vi "UI Initialize.vi"(8 "error in (no error)":errorcluster, 11 "New Project Wizard in":refnum<class "New Project Wizard.lvclass">) -> (0 "error out":errorcluster, 3 "New Project Wizard out":refnum<class "New Project Wizard.lvclass">)   [LabVIEW 2013, in "SET Project Editor.lvlib" / "New Project Wizard.lvclass"]
uses:
  New Project Wizard.lvclass
  New Project Wizard.lvclass/New Project Wizard.ctl
  UI Wizard/UI Wizard.lvclass
  SET Project Editor.lvlib
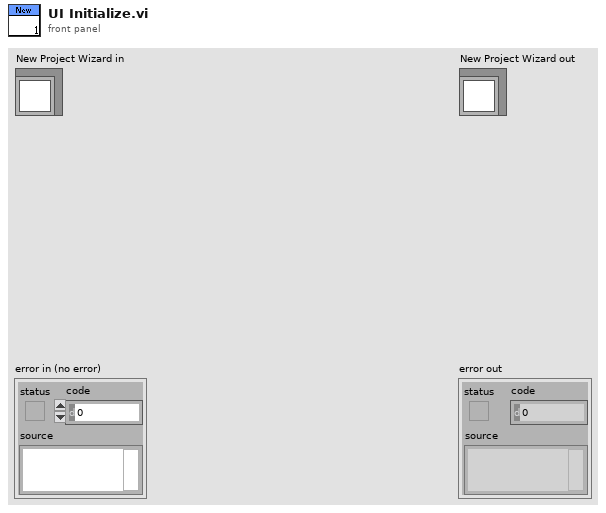
[diagram p1: front panel]
types:
  T1 = enum32{"Invalid", "Default", "Floating", "Floating/Auto-Hide", "Modal"}
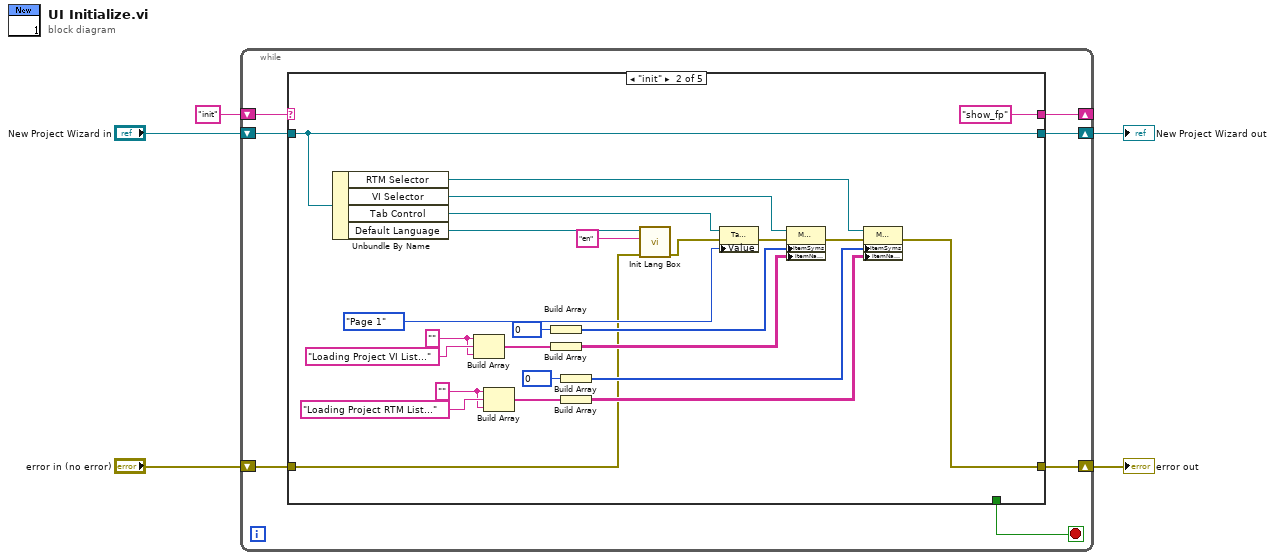
[diagram p0: block diagram]
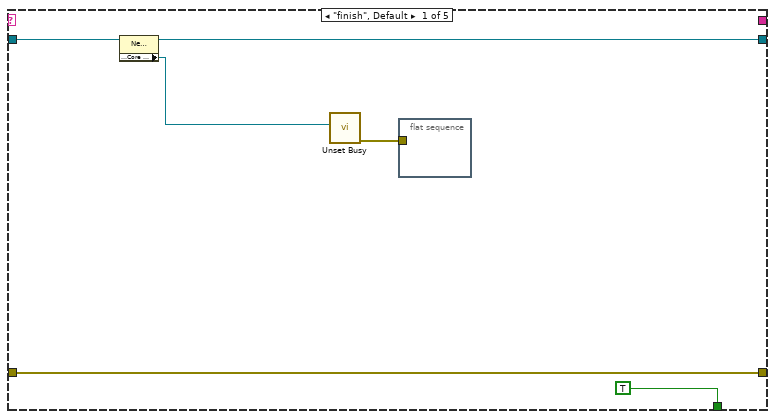
[diagram p2: hidden frame]
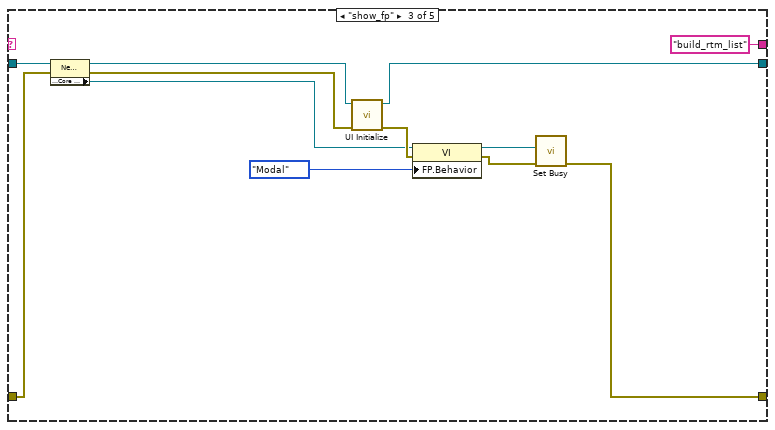
[diagram p3: hidden frame]
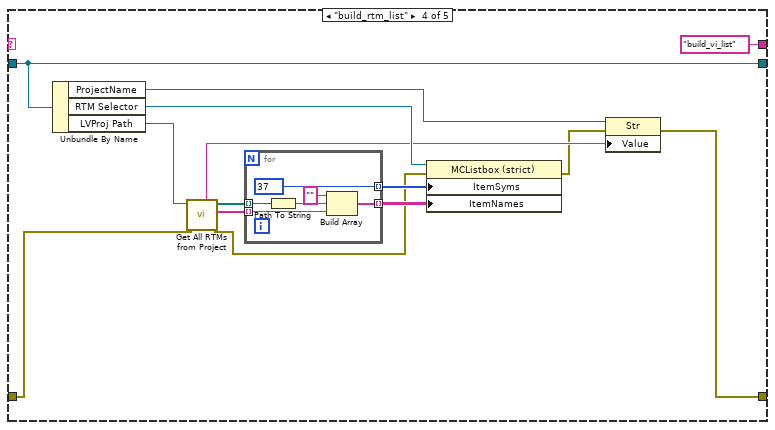
[diagram p4: hidden frame]
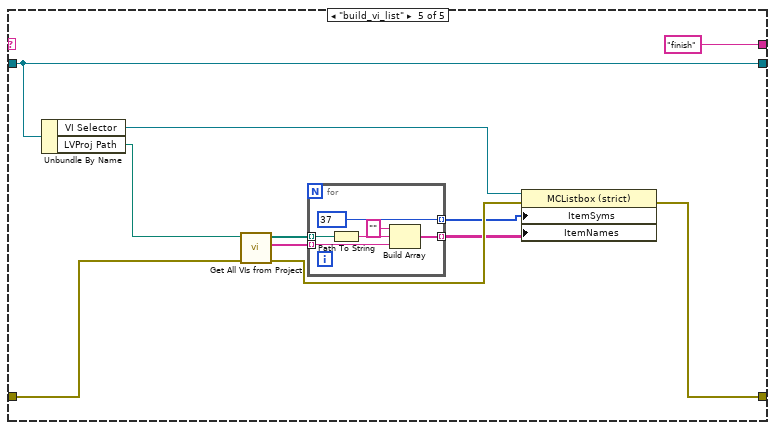
[diagram p5: hidden frame]
diagram:
  n1 = while {
    shift-right: [w8] -> w1
    shift-left: "New Project Wizard in" -> [w12]
    shift-right: [w7] -> _
    shift-left: "init" -> [w11]
    shift-right: [w9] -> w2
    shift-left: "error in (no error)" -> [w10]
    stop <- w6 stop-if-true
    n2 = case shown="\"init\"" w11 {
      tunnel: w12 -> [w16 w24 w53 w59 w77]
      tunnel: w10 -> [w18 w21 w50 w64 w78]
      tunnel: [w18 w25 w45 w57 w81] -> w9
      tunnel: [w15 w24 w48 w59 w77] -> w8
      tunnel: [_ "show_fp" "build_rtm_list" "build_vi_list" "finish"] -> w7
      tunnel: [TRUE _ _ _ _] -> w6
      frame "finish", Default {
        n3 = property class="New Project Wizard.lvclass"(reference=w16) -> (reference out=w15:refnum<class "New Project Wizard.lvclass">, "Properties:Core VI Refnum"=w14:refnum<vi>)  [unwired: 1 in, 1 out]
        n4 = call <vilib>:"Unset Busy.vi"("VI reference (current VI)"=w14) -> ("error out"=w17:errorcluster)  [unwired: 10 in]
        n5 = flat-sequence {
          tunnel: w17 -> [_]
          frame #0 {
          }
        }
      }
      frame "init" {
        w32 = ""
        w38 = ""
        n6 = Unbundle By Name(w24) -> ("RTM Selector"=w29:refnum<vi>, "VI Selector"=w37:refnum<vi>, "Tab Control"=w42:refnum<vi>, "Default Language"=w22:refnum<vi>)
        n7 = Build Array(w38, "Loading Project VI List...", w38) -> (w41:string[])
        n8 = Build Array(w32, "Loading Project RTM List...", w32) -> (w34:string[])
        n9 = Build Array(0) -> (w31:i32[])
        n10 = Build Array(w41) -> (w30:string[][])
        n11 = Build Array(0) -> (w28:i32[])
        n12 = Build Array(w34) -> (w27:string[][])
        n13 = call "Init Lang Box.vi"("error in (no error)"=w21, "Initial Value"="en", "ComboBox Ref in"=w22) -> ("error out"=w19:errorcluster)  [unwired: 7 in, 1 out]
        n14 = property class="TabCtl (strict)"(reference=w42, error in=w19, "Value"=enum32{"Page 1", "Page 2"}."Page 1") -> (error out=w36:errorcluster)  [unwired: 1 out]
        n15 = property on="Property Node" class="MCListbox (strict)"(reference=w37, error in=w36, "ItemSyms"=w31, "ItemNames"=w30) -> (error out=w26:errorcluster)  [unwired: 1 out]
        n16 = property on="Property Node" class="MCListbox (strict)"(reference=w29, error in=w26, "ItemSyms"=w28, "ItemNames"=w27) -> (error out=w25:errorcluster)  [unwired: 1 out]
      }
      frame "show_fp" {
        n17 = property class="New Project Wizard.lvclass"(reference=w53, error in=w50) -> (reference out=w51:refnum<class "New Project Wizard.lvclass">, error out=w49:errorcluster, "Properties:Core VI Refnum"=w52:refnum<vi>)
        n18 = call-parent "UI Initialize.vi"("error in (no error)"=w49, "UI Wizard in"=w51) -> ("error out"=w54:errorcluster, "UI Wizard out"=w48:refnum<class "New Project Wizard.lvclass">)  [unwired: 8 in]
        n19 = property class="VI"(reference=w52, error in=w54, "FP.Behavior"=T1."Modal" ("Front Panel Window:Behavior")) -> (reference out=w47:refnum<vi>, error out=w46:errorcluster)
        n20 = call <vilib>:"Set Busy.vi"("error in (no error)"=w46, "VI reference (current VI)"=w47) -> ("error out"=w45:errorcluster)  [unwired: 8 in, 1 out]
      }
      frame "build_rtm_list" {
        n21 = Unbundle By Name(w59) -> ("ProjectName"=w63:refnum<vi>, "RTM Selector"=w62:refnum<vi>, "LVProj Path"=w65:path)
        n22 = call "Get All RTMs from Project.vi"("error in (no error)"=w64, "Project Path"=w65) -> ("error out"=w61:errorcluster, "RTM Virtual Paths"=w67:string[], "Project RTMs"=w66:path[], "Project Name"=w60:string)  [unwired: 6 in]
        n23 = for {
          tunnel: w66 -> [w75] mode=indexing
          tunnel: w67 -> [w73] mode=indexing
          tunnel: [w71] -> w69 mode=indexing
          tunnel: [37] -> w68 mode=indexing
          n24 = Path To String(path=w75) -> (string=w74:string)
          n25 = Build Array("" ("element"), w74, w73) -> (w71:string[])
        }
        n26 = property on="Property Node" class="MCListbox (strict)"(reference=w62, error in=w61, "ItemSyms"=w68, "ItemNames"=w69) -> (error out=w58:errorcluster)  [unwired: 1 out]
        n27 = property class="Str"(reference=w63, error in=w58, "Value"=w60) -> (error out=w57:errorcluster)  [unwired: 1 out]
      }
      frame "build_vi_list" {
        n28 = Unbundle By Name(w77) -> ("VI Selector"=w80:refnum<vi>, "LVProj Path"=w79:path)
        n29 = call "Get All VIs from Project.vi"("error in (no error)"=w78, "Project Path"=w79) -> ("error out"=w86:errorcluster, "VI Virtual Paths"=w82:string[], "Project VIs"=w83:path[])  [unwired: 6 in, 1 out]
        n30 = for {
          tunnel: w83 -> [w92] mode=indexing
          tunnel: w82 -> [w90] mode=indexing
          tunnel: [w88] -> w85 mode=indexing
          tunnel: [37] -> w84 mode=indexing
          n31 = Path To String(path=w92) -> (string=w91:string)
          n32 = Build Array("" ("element"), w91, w90) -> (w88:string[])
        }
        n33 = property on="Property Node" class="MCListbox (strict)"(reference=w80, error in=w86, "ItemSyms"=w84, "ItemNames"=w85) -> (error out=w81:errorcluster)  [unwired: 1 out]
      }
    }
  }
  "error out" <- w2
  "New Project Wizard out" <- w1
